vi "2.1 Interpret NMEA Sentence.vi"(11 "NMEA Sentence":string) -> ()   [LabVIEW 2011]
doc: "Interprets the NMEA 0813 sentences that we are using from our Airmar PB200 WeatherStation sensor.\nBy Jaime McCandless\nTODO: finish implementing NMEA sentences"
uses:
  2 Typedefs/Velocity.ctl
  2 Typedefs/apparent wind.ctl
  2 Typedefs/pitch and roll.ctl
  2 Globals/2 Global.vi
  <vilib>/regexp/Match Regular Expression.xnode
panel:
  out "Heading":dbl
  in  "UTC Time Zone":i32=-5
  out "Tab Control":T1(tab)
  out "GPS (GGA) Data":T2
  out "GPS (GLL) Data":T3
  out "UTC Time":timestamp
  out "Local Time":timestamp
  out "Lattitude (ddmm.mmmm)":dbl format="%_8g"
  out "Lattitude North/South":string
  out "Longitude (ddmm.mmmm)":dbl format="%_8g"
  out "Longitude East/West":string
  out "Speed over ground (knots)":dbl format="%_3g"
  out "Course over ground (degrees)":dbl format="%_4g"
  out "Magnetic Variation (degrees)":dbl format="%_4g"
  out "Variation East/West":string
  out "GPS (RMC) Data":T4 {"Course over ground (degrees)" format="%#.6g"; "Speed over ground (knots)" format="%#.6g"; "Magnetic Variation (degrees)" format="%#.6g"; "Longitude (ddmm.mmmm)" format="%#.6g"; "Lattitude (ddmm.mmmm)" format="%#.6g"}
  out "GPS Data Valid?":bool
  out "GPS (VTG) Data":T5
  out "Turn (ROT) Data":T6
  out "Wind (MWV) Data":T7
  out "Transducer (XDR) B Data":cluster{"Pitch (deg)":dbl, "Roll (deg)":dbl}
  out "Transducer (XDR) A Data":T8
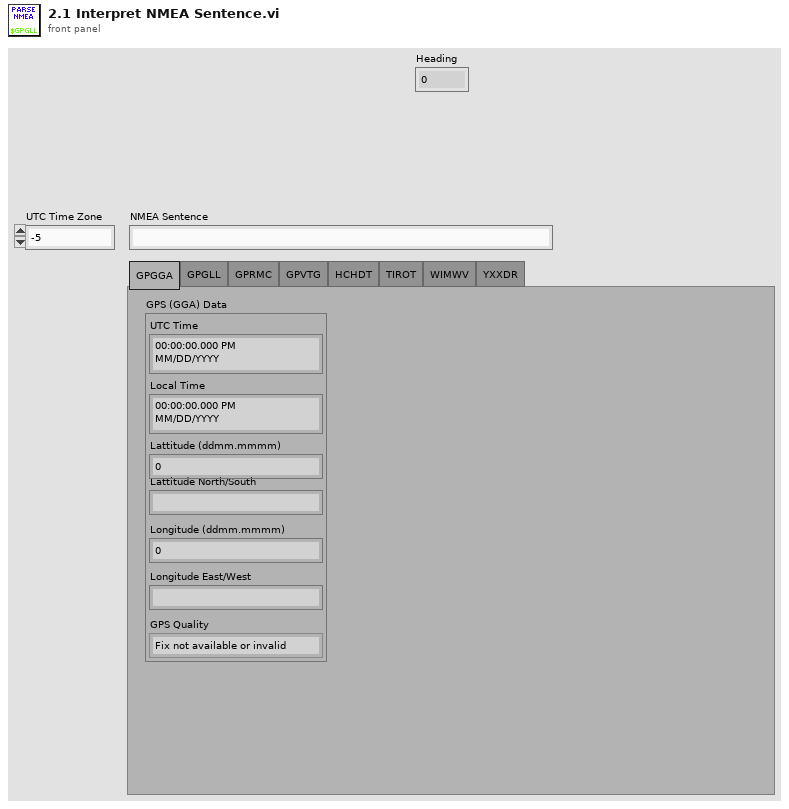
[diagram p1: front panel]
types:
  T1 = enum32{"GPGGA", "GPGLL", "GPRMC", "GPVTG", "HCHDT", "TIROT", "WIMWV", "YXXDR"}
  T2 = cluster{"UTC Time":timestamp, "Local Time":timestamp, "Lattitude (ddmm.mmmm)":dbl, "Lattitude North/South":string, "Longitude (ddmm.mmmm)":dbl, "Longitude East/West":string, "GPS Quality":enum16{"Fix not available or invalid", "GPS SPS Mode, fix valid", "Differential GPS, SPS Mode, fix valid", "GPS PPS Mode, fix valid", "Real Time Kinematic (RTK)", "Float RTK", "Estimated (dead reckoning) Mode", "Manual Input Mode", "Simulator Mode"}}
  T3 = cluster{"UTC Time":timestamp, "Local Time":timestamp, "Lattitude (ddmm.mmmm)":dbl, "Lattitude North/South":string, "Longitude (ddmm.mmmm)":dbl, "Longitude East/West":string, "GPS Mode":string, "GPS Data Valid?":bool}
  T4 = cluster{"UTC Time":timestamp, "Local Time":timestamp, "Lattitude (ddmm.mmmm)":dbl, "Lattitude North/South":string, "Longitude (ddmm.mmmm)":dbl, "Longitude East/West":string, "Magnetic Variation (degrees)":dbl, "Variation East/West":string, "Speed over ground (knots)":dbl, "Course over ground (degrees)":dbl}
  T5 = cluster{"Course Over Ground (True)":dbl, "Course Over Ground (Magnetic)":dbl, "Speed Over Ground (Knots)":dbl, "Speed Over Ground (km/hr)":dbl, "GPS Mode":string}
  T6 = cluster{"Rate of Turn (deg/min)":dbl, "Turn Rotation Data Valid?":bool}
  T7 = cluster{"Angle relative to boat (deg)":dbl, "Wind Data Valid?":bool, "Wind speed (knots)":dbl, "True (T) or Relative (R)":string}
  T8 = cluster{"Calc. Relative Wind Chill (degC)":dbl, "Calc. Theoretical Wind Chill (degC)":dbl, "Calc. Heat Index (degC)":dbl, "Meas. Barometric Pressure (bars)":dbl}
  T9 = cluster{"second":i32, "minute":i32, "hour":i32, "day of month":i32, "month":i32, "year":i32, "day of week":i32, "day of year":i32, "is DST":i32}
  T10 = typedef "Velocity.ctl" = cluster{"East":dbl, "North":dbl}
  T11 = typedef "apparent wind.ctl" = cluster{"Toward Fore":dbl, "Toward Starboard":dbl}
  T12 = typedef "pitch and roll.ctl" = cluster{"Pitch":dbl, "Roll":dbl}
  T13 = typedef "UTM Location.ctl" = cluster{"UTM Zone":dbl, "Hemisphere":enum16{"North", "South"}, "East":dbl, "North":dbl}
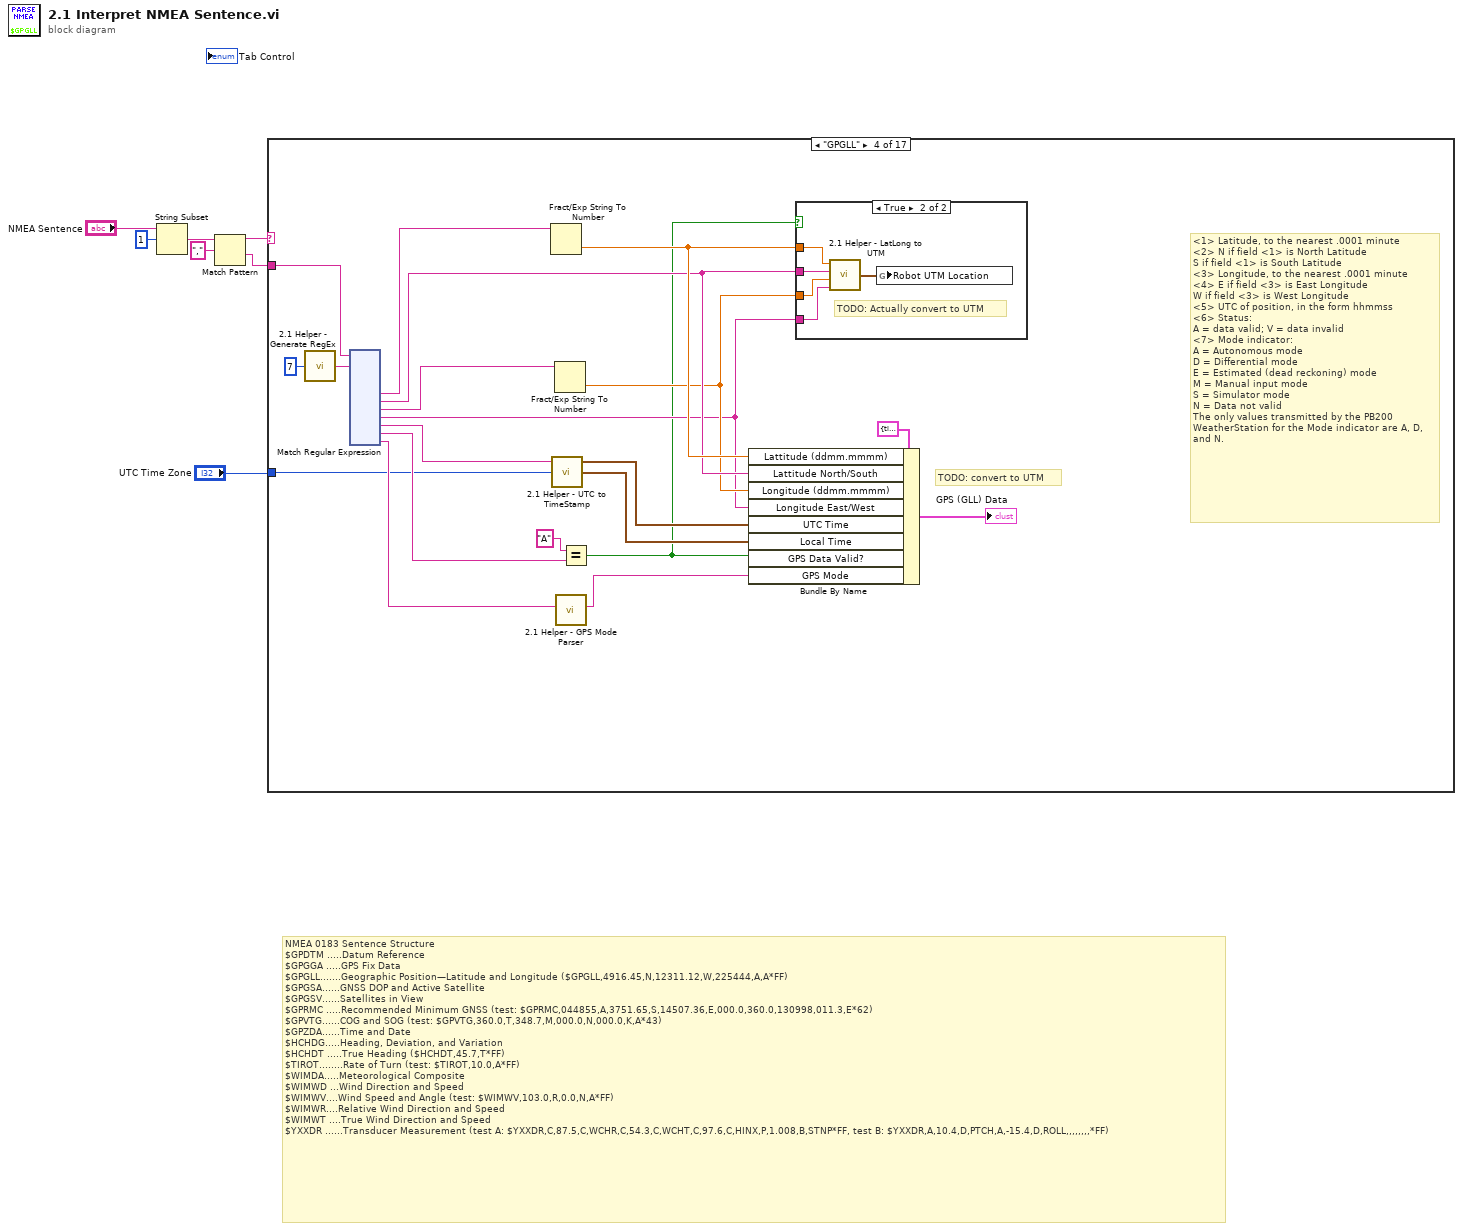
[diagram p0: block diagram]
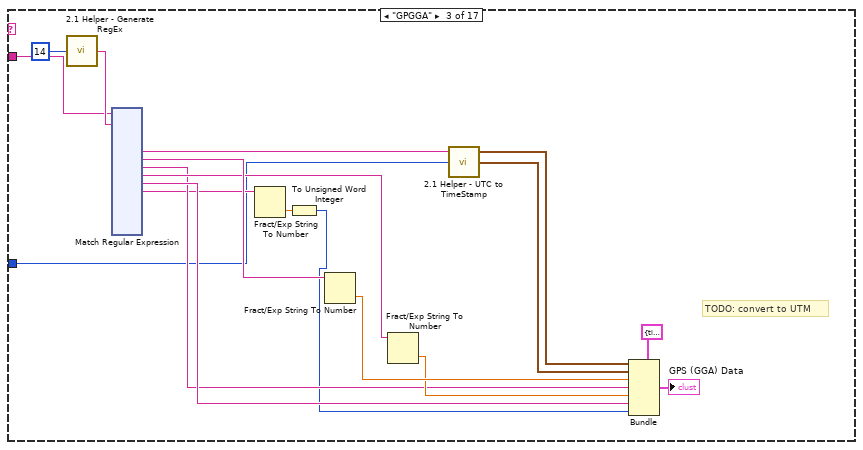
[diagram p4: hidden frame]
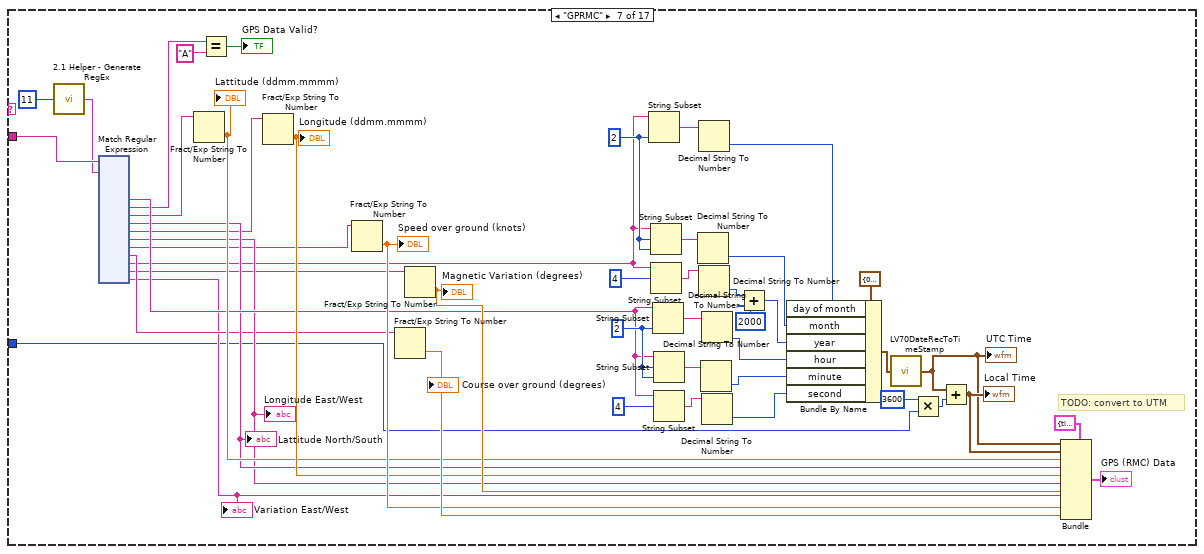
[diagram p8: hidden frame]
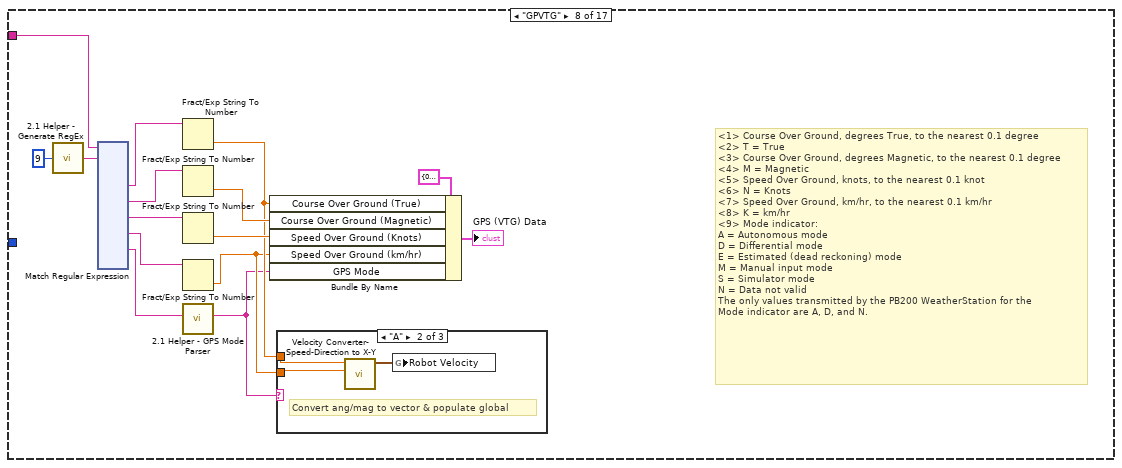
[diagram p9: hidden frame]
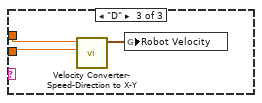
[diagram p11: hidden frame]
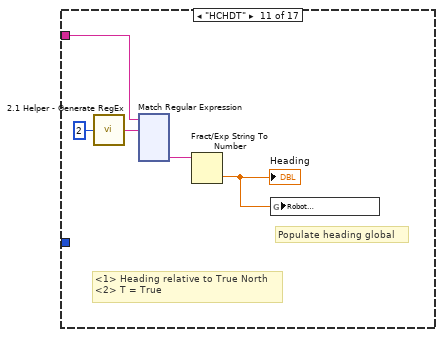
[diagram p14: hidden frame]
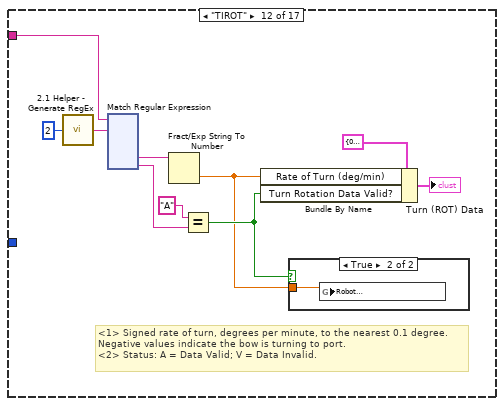
[diagram p15: hidden frame]
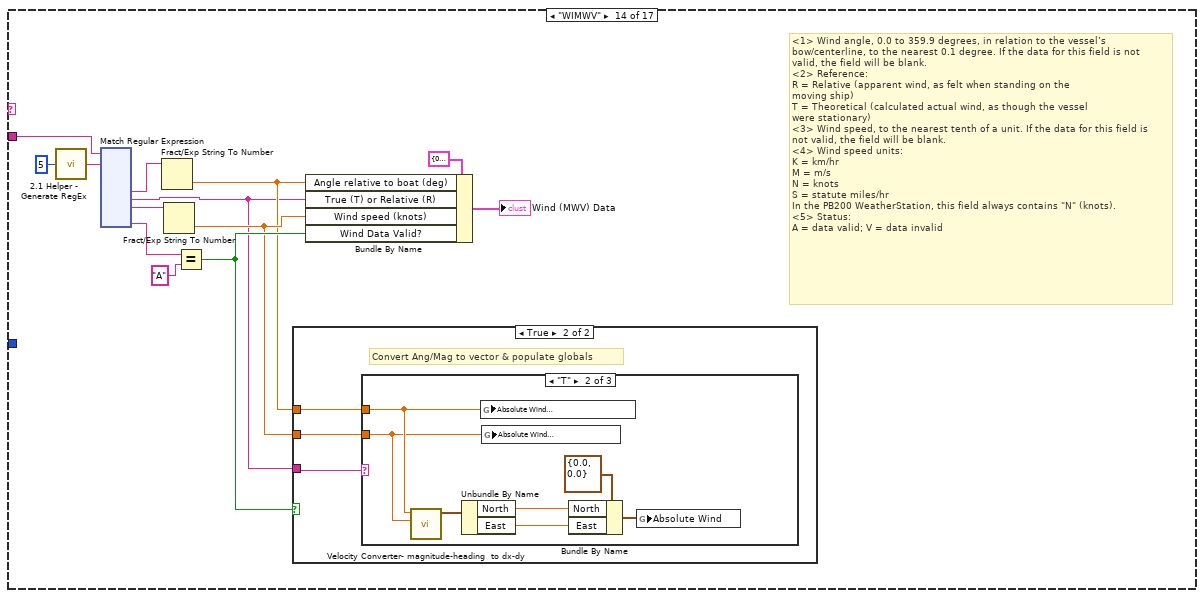
[diagram p18: hidden frame]
diagram:
  # "NMEA 0183 Sentence Structure\n$GPDTM .....Datum Reference\n$GPGGA .....GPS Fix Data\n$GPGLL.......Geographic Position—Latitude and Longitude ($GPGLL,4916.45,N,12311.12,W,225444,A,A*FF)\n$GPGSA......GNSS DOP and Active Satellite\n$GPGSV......Satellites in View\n$GPRMC .....Recommended Minimum GNSS (test: $GPRMC,044855,A,3751.65,S,14507.36,E,000.0,360.0,130998,011.3,E*62)\n$GPVTG......COG and SOG (test: $GPVTG,360.0,T,348.7,M,000.0,N,000.0,K,A*43)\n$GPZDA......Time and Date\n$HCHDG.....Heading, Deviation, and Variation\n$HCHDT .....True Heading ($HCHDT,45.7,T*FF)\n$TIROT........Rate of Turn (test: $TIROT,10.0,A*FF)\n$WIMDA.....Meteorological Composite\n$WIMWD ...Wind Direction and Speed\n$WIMWV....Wind Speed and Angle (test: $WIMWV,103.0,R,0.0,N,A*FF)\n$WIMWR....Relative Wind Direction and Speed\n$WIMWT ....True Wind Direction and Speed\n$YXXDR ......Transducer Measurement (test A: $YXXDR,C,87.5,C,WCHR,C,54.3,C,WCHT,C,97.6,C,HINX,P,1.008,B,STNP*FF, test B: $YXXDR,A,10.4,D,PTCH,A,-15.4,D,ROLL,,,,,,,,*FF)"
  n1 = String Subset(string="NMEA Sentence", offset (0)=1) -> (substring=w4:string)  [unwired: 1 in]
  n2 = Match Pattern(string=w4, regular expression=",") -> (before substring=w5:string, after substring=w6:string)  [unwired: 1 in, 2 out]
  n3 = case shown="\"GPGLL\"" w5 {
    tunnel: w6 -> [_ _ w23 w163 _ _ w307 w476 _ _ w610 w732 _ w859 _ _ w1003]
    tunnel: "UTC Time Zone" -> [_ _ w8 w155 _ _ w293 _ _ _ _ _ _ _ _ _ _]
    frame "", Default {
    }
    frame "GPDTM" {
    }
    frame "GPGGA" {
      # "TODO: convert to UTM"
      n4 = call "2.1 Helper - Generate RegEx.vi"("# Datums"=14) -> ("RegEx"=w24:string)
      n5 = xnode "Match Regular Expression"("input string"=w23, "regular expression"=w24) -> ("submatch 1"=w11:string, "submatch 2"=w19:string, "submatch 3"=w16:string, "submatch 4"=w18:string, "submatch 5"=w17:string, "submatch 6"=w15:string)  [unwired: 4 in, 10 out]
      n6 = Fract/Exp String To Number(string=w15) -> (number=w14:dbl)  [unwired: 3 in, 1 out]
      n7 = To Unsigned Word Integer(number=w14) -> (unsigned 16bit integer=w13:u16)
      n8 = Fract/Exp String To Number(string=w19) -> (number=w22:dbl)  [unwired: 3 in, 1 out]
      n9 = Fract/Exp String To Number(string=w18) -> (number=w21:dbl)  [unwired: 3 in, 1 out]
      n10 = call "2.1 Helper - UTC to TimeStamp.vi"("UTC Time Zone in"=w8, "UTC (hhmmss)"=w11) -> ("Local Time"=w9:timestamp, "UTC Time"=w10:timestamp)  [unwired: 2 in]
      n11 = Bundle(cluster=T2 {"UTC Time"=timestamp(0 s since 1904-01-01), "Local Time"=timestamp(0 s since 1904-01-01), "Lattitude (ddmm.mmmm)"=0.0, "Lattitude North/South"="", "Longitude (ddmm.mmmm)"=0.0, "Longitude East/West"="", "GPS Quality"=enum."GPS SPS Mode, fix valid"} ("Cluster"), "UTC Time"=w10, "Local Time"=w9, "Lattitude (ddmm.mmmm)"=w22, "Lattitude North/South"=w16, "Longitude (ddmm.mmmm)"=w21, "Longitude East/West"=w17, "GPS Quality"=w13) -> (→"GPS (GGA) Data":T2)
    }
    frame "GPGLL" {
      # "<1> Latitude, to the nearest .0001 minute\n<2> N if field <1> is North Latitude\nS if field <1> is South Latitude\n<3> Longitude, to the nearest .0001 minute\n<4> E if field <3> is East Longitude\nW if field <3> is West Longitude\n<5> UTC of position, in the form hhmmss\n<6> Status:\nA = data valid; V = data invalid\n<7> Mode indicator:\nA = Autonomous mode\nD = Differential mode\nE = Estimated (dead reckoning) mode\nM = Manual input mode\nS = Simulator mode\nN = Data not valid\nThe only values transmitted by the PB200 WeatherStation for the Mode indicator are A, D, and N."
      # "TODO: convert to UTM"
      n12 = call "2.1 Helper - Generate RegEx.vi"("# Datums"=7) -> ("RegEx"=w167:string)
      n13 = xnode "Match Regular Expression"("input string"=w163, "regular expression"=w167) -> ("submatch 1"=w166:string, "submatch 2"=w152:string, "submatch 3"=w165:string, "submatch 4"=w150:string, "submatch 5"=w162:string, "submatch 6"=w158:string, "submatch 7"=w164:string)  [unwired: 4 in, 5 out]
      n14 = Fract/Exp String To Number(string=w166) -> (number=w153:dbl)  [unwired: 3 in, 1 out]
      n15 = call "2.1 Helper - UTC to TimeStamp.vi"("UTC Time Zone in"=w155, "UTC (hhmmss)"=w162) -> ("Local Time"=w157:timestamp, "UTC Time"=w156:timestamp)  [unwired: 2 in]
      n16 = Fract/Exp String To Number(string=w165) -> (number=w151:dbl)  [unwired: 3 in, 1 out]
      n17 = call "2.1 Helper - GPS Mode Parser.vi"("GPS Mode (Char)"=w164) -> ("GPS Mode (Description)"=w160:string)  [unwired: 6 in]
      n18 = Equal?(x="A" ("y"), y=w158) -> (x = y?=w149:bool)
      n19 = Bundle By Name(cluster=T3 {"UTC Time"=timestamp(0 s since 1904-01-01), "Local Time"=timestamp(0 s since 1904-01-01), "Lattitude (ddmm.mmmm)"=0.0, "Lattitude North/South"="", "Longitude (ddmm.mmmm)"=0.0, "Longitude East/West"="", "GPS Mode"="", "GPS Data Valid?"=FALSE} ("Cluster"), "Lattitude (ddmm.mmmm)"=w153, "Lattitude North/South"=w152, "Longitude (ddmm.mmmm)"=w151, "Longitude East/West"=w150, "UTC Time"=w156, "Local Time"=w157, "GPS Data Valid?"=w149, "GPS Mode"=w160) -> (→"GPS (GLL) Data":T3)
      n20 = case shown="True" w149 {
        tunnel: w153 -> [_ w172]
        tunnel: w152 -> [_ w171]
        tunnel: w151 -> [_ w170]
        tunnel: w150 -> [_ w169]
        frame False {
        }
        frame True {
          # "TODO: Actually convert to UTM"
          n21 = call "2.1 Helper - LatLong to UTM.vi"("East/West"=w169, "Longitude"=w170, "North/South"=w171, "Latitude"=w172) -> ("Robot UTM Location"=w173:T13)
          n22 = global write "2 Global.vi" "Robot UTM Location"(w173) -> ()
        }
      }
    }
    frame "GPGSA" {
    }
    frame "GPGSV" {
    }
    frame "GPRMC" {
      w325 = 2 ("length (rest)")
      w315 = 2 ("length (rest)")
      # "TODO: convert to UTM"
      n23 = call "2.1 Helper - Generate RegEx.vi"("# Datums"=11) -> ("RegEx"=w295:string)
      n24 = xnode "Match Regular Expression"("input string"=w307, "regular expression"=w295) -> ("submatch 1"=w306:string, "submatch 2"=w305:string, "submatch 3"=w304:string, "submatch 4"=w303:string, "submatch 5"=w302:string, "submatch 6"=w301:string, "submatch 7"=w300:string, "submatch 8"=w299:string, "submatch 9"=w298:string, "submatch 10"=w297:string, "submatch 11"=w296:string)  [unwired: 4 in, 5 out]
      "Lattitude North/South" <- w303
      "Longitude East/West" <- w301
      "Variation East/West" <- w296
      n25 = Fract/Exp String To Number(string=w304) -> (number=w334:dbl)  [unwired: 3 in, 1 out]
      "Lattitude (ddmm.mmmm)" <- w334
      n26 = Equal?(x=w305, y="A") -> (x = y?=→"GPS Data Valid?":bool)
      n27 = Fract/Exp String To Number(string=w302) -> (number=w335:dbl)  [unwired: 3 in, 1 out]
      "Longitude (ddmm.mmmm)" <- w335
      n28 = Fract/Exp String To Number(string=w300) -> (number=w337:dbl)  [unwired: 3 in, 1 out]
      "Speed over ground (knots)" <- w337
      n29 = Fract/Exp String To Number(string=w299) -> (number=w338:dbl)  [unwired: 3 in, 1 out]
      "Course over ground (degrees)" <- w338
      n30 = Fract/Exp String To Number(string=w297) -> (number=w336:dbl)  [unwired: 3 in, 1 out]
      "Magnetic Variation (degrees)" <- w336
      n31 = String Subset(string=w298, length (rest)=w325) -> (substring=w326:string)  [unwired: 1 in]
      n32 = String Subset(string=w298, offset (0)=w325, length (rest)=w325) -> (substring=w324:string)
      n33 = String Subset(string=w298, offset (0)=4) -> (substring=w322:string)  [unwired: 1 in]
      n34 = String Subset(string=w306, length (rest)=w315) -> (substring=w311:string)  [unwired: 1 in]
      n35 = String Subset(string=w306, offset (0)=w315, length (rest)=w315) -> (substring=w317:string)
      n36 = String Subset(string=w306, offset (0)=4) -> (substring=w319:string)  [unwired: 1 in]
      n37 = Decimal String To Number(string=w324) -> (number=w328:i32)  [unwired: 2 in, 1 out]
      n38 = Decimal String To Number(string=w326) -> (number=w327:i32)  [unwired: 2 in, 1 out]
      n39 = Decimal String To Number(string=w322) -> (number=w329:i32)  [unwired: 2 in, 1 out]
      n40 = Decimal String To Number(string=w317) -> (number=w316:i32)  [unwired: 2 in, 1 out]
      n41 = Decimal String To Number(string=w311) -> (number=w314:i32)  [unwired: 2 in, 1 out]
      n42 = Decimal String To Number(string=w319) -> (number=w320:i32)  [unwired: 2 in, 1 out]
      n43 = Add(x=w329, y=2000) -> (x+y=w331:i32)
      n44 = Bundle By Name(cluster=T9 {"second"=0, "minute"=0, "hour"=0, "day of month"=0, "month"=0, "year"=0, "day of week"=0, "day of year"=0, "is DST"=0} ("date time rec"), "day of month"=w327, "month"=w328, "year"=w331, "hour"=w314, "minute"=w316, "second"=w320) -> (w312:T9)
      n45 = call <vilib>:"LV70DateRecToTimeStamp.vi"("date time rec"=w312) -> ("Time Stamp"=w332:timestamp)
      "UTC Time" <- w332
      n46 = Multiply(x=3600 ("number"), y=w293) -> (x*y=w294:i32)
      n47 = Add(x=w332, y=w294) -> (x+y=w333:timestamp)
      "Local Time" <- w333
      n48 = Bundle(cluster=T4 {"UTC Time"=timestamp(0 s since 1904-01-01), "Local Time"=timestamp(0 s since 1904-01-01), "Lattitude (ddmm.mmmm)"=0.0, "Lattitude North/South"="", "Longitude (ddmm.mmmm)"=0.0, "Longitude East/West"="", "Magnetic Variation (degrees)"=0.0, "Variation East/West"="", "Speed over ground (knots)"=0.0, "Course over ground (degrees)"=0.0} ("Cluster"), "UTC Time"=w332, "Local Time"=w333, "Lattitude (ddmm.mmmm)"=w334, "Lattitude North/South"=w303, "Longitude (ddmm.mmmm)"=w335, "Longitude East/West"=w301, "Magnetic Variation (degrees)"=w336, "Variation East/West"=w296, "Speed over ground (knots)"=w337, "Course over ground (degrees)"=w338) -> (→"GPS (RMC) Data":T4)
    }
    frame "GPVTG" {
      # "<1> Course Over Ground, degrees True, to the nearest 0.1 degree\n<2> T = True\n<3> Course Over Ground, degrees Magnetic, to the nearest 0.1 degree\n<4> M = Magnetic\n<5> Speed Over Ground, knots, to the nearest 0.1 knot\n<6> N = Knots\n<7> Speed Over Ground, km/hr, to the nearest 0.1 km/hr\n<8> K = km/hr\n<9> Mode indicator:\nA = Autonomous mode\nD = Differential mode\nE = Estimated (dead reckoning) mode\nM = Manual input mode\nS = Simulator mode\nN = Data not valid\nThe only values transmitted by the PB200 WeatherStation for the\nMode indicator are A, D, and N."
      n49 = call "2.1 Helper - Generate RegEx.vi"("# Datums"=9) -> ("RegEx"=w477:string)
      n50 = xnode "Match Regular Expression"("input string"=w476, "regular expression"=w477) -> ("submatch 1"=w473:string, "submatch 3"=w472:string, "submatch 5"=w470:string, "submatch 7"=w468:string, "submatch 9"=w467:string)  [unwired: 4 in, 11 out]
      n51 = Fract/Exp String To Number(string=w473) -> (number=w466:dbl)  [unwired: 3 in, 1 out]
      n52 = Fract/Exp String To Number(string=w472) -> (number=w471:dbl)  [unwired: 3 in, 1 out]
      n53 = Fract/Exp String To Number(string=w470) -> (number=w469:dbl)  [unwired: 3 in, 1 out]
      n54 = Fract/Exp String To Number(string=w468) -> (number=w465:dbl)  [unwired: 3 in, 1 out]
      n55 = call "2.1 Helper - GPS Mode Parser.vi"("GPS Mode (Char)"=w467) -> ("GPS Mode (Description)"=w464:string)  [unwired: 6 in]
      n56 = Bundle By Name(cluster=T5 {"Course Over Ground (True)"=0.0, "Course Over Ground (Magnetic)"=0.0, "Speed Over Ground (Knots)"=0.0, "Speed Over Ground (km/hr)"=0.0, "GPS Mode"=""} ("GPS (VTG) Data 2"), "Course Over Ground (True)"=w466, "Course Over Ground (Magnetic)"=w471, "Speed Over Ground (Knots)"=w469, "Speed Over Ground (km/hr)"=w465, "GPS Mode"=w464) -> (→"GPS (VTG) Data":T5)
      n57 = case shown="\"A\"" w464 {
        tunnel: w466 -> [_ w481 w484]
        tunnel: w465 -> [_ w480 w483]
        frame "N", Default {
          # "Data not valid"
        }
        frame "A" {
          # "Convert ang/mag to vector & populate global"
          n58 = call "Velocity Converter- Speed-Direction to X-Y.vi"("Speed"=w480, "Heading"=w481) -> ("Velocity Out"=w479:T10)  [unwired: 9 in]
          n59 = global write "2 Global.vi" "Robot Velocity"(w479) -> ()
        }
        frame "D" {
          n60 = call "Velocity Converter- Speed-Direction to X-Y.vi"("Speed"=w483, "Heading"=w484) -> ("Velocity Out"=w482:T10)  [unwired: 9 in]
          n61 = global write "2 Global.vi" "Robot Velocity"(w482) -> ()
        }
      }
    }
    frame "GPZDA" {
    }
    frame "HCHDG " {
    }
    frame "HCHDT" {
      # "Populate heading global"
      # "<1> Heading relative to True North\n<2> T = True"
      n62 = call "2.1 Helper - Generate RegEx.vi"("# Datums"=2) -> ("RegEx"=w611:string)
      n63 = xnode "Match Regular Expression"("input string"=w610, "regular expression"=w611) -> ("submatch 1"=w609:string)  [unwired: 4 in, 5 out]
      n64 = Fract/Exp String To Number(string=w609) -> (number=w608:dbl)  [unwired: 3 in, 1 out]
      "Heading" <- w608
      n65 = global write "2 Global.vi" "Robot\nHeading"(w608) -> ()
    }
    frame "TIROT" {
      # "<1> Signed rate of turn, degrees per minute, to the nearest 0.1 degree.\nNegative values indicate the bow is turning to port.\n<2> Status: A = Data Valid; V = Data Invalid."
      n66 = call "2.1 Helper - Generate RegEx.vi"("# Datums"=2) -> ("RegEx"=w734:string)
      n67 = xnode "Match Regular Expression"("input string"=w732, "regular expression"=w734) -> ("submatch 1"=w733:string, "submatch 2"=w728:string)  [unwired: 4 in, 5 out]
      n68 = Fract/Exp String To Number(string=w733) -> (number=w726:dbl)  [unwired: 3 in, 1 out]
      n69 = Equal?(x="A" ("y"), y=w728) -> (x = y?=w727:bool)
      n70 = Bundle By Name(cluster=T6 {"Rate of Turn (deg/min)"=0.0, "Turn Rotation Data Valid?"=TRUE} ("Turn (ROT) Data 2"), "Rate of Turn (deg/min)"=w726, "Turn Rotation Data Valid?"=w727) -> (→"Turn (ROT) Data":T6)
      n71 = case shown="True" w727 {
        tunnel: w726 -> [_ w736]
        frame False {
        }
        frame True {
          n72 = global write "2 Global.vi" "Robot\nRate of Turn"(w736) -> ()
        }
      }
    }
    frame "WIMDA" {
    }
    frame "WIMWV" {
      # "<1> Wind angle, 0.0 to 359.9 degrees, in relation to the vessel’s\nbow/centerline, to the nearest 0.1 degree. If the data for this field is not\nvalid, the field will be blank.\n<2> Reference:\nR = Relative (apparent wind, as felt when standing on the\nmoving ship)\nT = Theoretical (calculated actual wind, as though the vessel\nwere stationary)\n<3> Wind speed, to the nearest tenth of a unit. If the data for this field is\nnot valid, the field will be blank.\n<4> Wind speed units:\nK = km/hr\nM = m/s\nN = knots\nS = statute miles/hr\nIn the PB200 WeatherStation, this field always contains \"N\" (knots).\n<5> Status:\nA = data valid; V = data invalid"
      n73 = call "2.1 Helper - Generate RegEx.vi"("# Datums"=5) -> ("RegEx"=w862:string)
      n74 = xnode "Match Regular Expression"("input string"=w859, "regular expression"=w862) -> ("submatch 1"=w861:string, "submatch 2"=w851:string, "submatch 3"=w856:string, "submatch 5"=w855:string)  [unwired: 4 in, 6 out]
      n75 = Fract/Exp String To Number(string=w861) -> (number=w852:dbl)  [unwired: 3 in, 1 out]
      n76 = Fract/Exp String To Number(string=w856) -> (number=w853:dbl)  [unwired: 3 in, 1 out]
      n77 = Equal?(x=w855, y="A") -> (x = y?=w854:bool)
      n78 = case shown="True" w854 {
        tunnel: w853 -> [_ w866]
        tunnel: w852 -> [_ w865]
        tunnel: w851 -> [_ w864]
        frame False {
        }
        frame True {
          # "Convert Ang/Mag to vector & populate globals"
          n79 = case shown="\"T\"" w864 {
            tunnel: w866 -> [_ w868 w874]
            tunnel: w865 -> [_ w869 w875]
            frame "\u0000", Default {
            }
            frame "T" {
              n80 = call "Velocity Converter- magnitude-heading  to dx-dy.vi"("Magnitude"=w868, "Heading"=w869) -> ("Vector Out"=w873:T10)  [unwired: 9 in]
              n81 = Unbundle By Name(w873) -> ("North"=w871:dbl, "East"=w870:dbl)
              n82 = global write "2 Global.vi" "Absolute Wind\nDirection"(w869) -> ()
              n83 = global write "2 Global.vi" "Absolute Wind\nSpeed"(w868) -> ()
              n84 = Bundle By Name(cluster=T10 {"East"=0.0, "North"=0.0} ("Absolute Wind"), "North"=w871, "East"=w870) -> (w872:T10)
              n85 = global write "2 Global.vi" "Absolute Wind"(w872) -> ()
            }
            frame "R" {
              n86 = call "Velocity Converter- magnitude-heading  to dx-dy.vi"("Magnitude"=w874, "Heading"=w875) -> ("Vector Out"=w876:T10)  [unwired: 9 in]
              n87 = Unbundle By Name(w876) -> ("North"=w879:dbl, "East"=w880:dbl)
              n88 = global write "2 Global.vi" "Apparent Wind\nDirection"(w875) -> ()
              n89 = global write "2 Global.vi" "Apparent Wind\nSpeed"(w874) -> ()
              n90 = Bundle By Name(cluster=T11 {"Toward Fore"=0.0, "Toward Starboard"=0.0} ("Apparent Wind"), "Toward Fore"=w879, "Toward Starboard"=w880) -> (w878:T11)
              n91 = global write "2 Global.vi" "Apparent Wind"(w878) -> ()
            }
          }
        }
      }
      n92 = Bundle By Name(cluster=T7 {"Angle relative to boat (deg)"=0.0, "Wind Data Valid?"=TRUE, "Wind speed (knots)"=0.0, "True (T) or Relative (R)"=""} ("Wind (MWV) Data 2"), "Angle relative to boat (deg)"=w852, "True (T) or Relative (R)"=w851, "Wind speed (knots)"=w853, "Wind Data Valid?"=w854) -> (→"Wind (MWV) Data":T7)
    }
    frame "WIMWR" {
    }
    frame "WIMWT" {
    }
    frame "YXXDR" {
      n93 = call "2.1 Helper - Generate RegEx.vi"("# Datums"=16) -> ("RegEx"=w1005:string)
      n94 = xnode "Match Regular Expression"("input string"=w1003, "regular expression"=w1005) -> ("submatch 1"=w1002:string, "submatch 2"=w1001:string, "submatch 6"=w1000:string, "submatch 10"=w999:string, "submatch 14"=w998:string)  [unwired: 4 in, 16 out]
      n95 = case shown="\"C\"" w1002 {
        tunnel: w1001 -> [_ w1011 w1021]
        tunnel: w1000 -> [_ w1010 w1020]
        tunnel: w999 -> [_ _ w1018]
        tunnel: w998 -> [_ _ w1019]
        frame "", Default {
        }
        frame "A" {
          # "TYPE B:\n<1> A = angular displacement\n<2> Pitch: oscillation of vessel about its latitudinal axis. Bow moving up is positive. Value reported to the nearest 0.1 degree.\n<3> D = degrees\n<4> PTCH (ID indicating pitch of vessel)\n<5> A = angular displacement\n<6> Roll: oscillation of vessel about its longitudinal axis. Roll to the starboard is positive. Value reported to the nearest 0.1 degree.\n<7> D = degrees\n<8> ROLL (ID indicating roll of vessel)\n<9> Not used\n<10> Not used\n<11> Not used\n<12> Not used\n<13> Not used\n<14> Not used\n<15> Not used\n<16> Not used"
          n96 = Fract/Exp String To Number(string=w1011) -> (number=w1007:dbl)  [unwired: 3 in, 1 out]
          n97 = Fract/Exp String To Number(string=w1010) -> (number=w1006:dbl)  [unwired: 3 in, 1 out]
          n98 = Bundle By Name(cluster=cluster{"Pitch (deg)":dbl, "Roll (deg)":dbl} {"Pitch (deg)"=103.0, "Roll (deg)"=103.0} ("Transducer (XDR) B Data 2"), "Pitch (deg)"=w1007, "Roll (deg)"=w1006) -> (→"Transducer (XDR) B Data":cluster{"Pitch (deg)":dbl, "Roll (deg)":dbl})
          n99 = Bundle By Name(cluster=T12 {"Pitch"=0.0, "Roll"=0.0} ("Robot Pitch/Roll"), "Pitch"=w1007, "Roll"=w1006) -> (w1008:T12)
          n100 = global write "2 Global.vi" "Robot Pitch/Roll"(w1008) -> ()
        }
        frame "C" {
          # "TYPE A:\n<1> C = temperature\n<2> Calculated “relative” wind chill temperature, degrees Celsius, to the nearest 0.1 degree\n<3> C = degrees C\n<4> WCHR (ID indicating relative wind chill)\n<5> C = temperature\n<6> Calculated “theoretical” wind chill temperature, degrees Celsius, to the nearest 0.1 degree\n<7> C = degrees C\n<8> WCHT (ID indicating theoretical wind chill)\n<9> C = temperature\n<10> Calculated heat index, degrees Celsius, to the nearest 0.1 degree (this field left blank by WeatherStation)\n<11> C = degrees C\n<12> HINX (ID indicating heat index)\n<13> P = pressure\n<14> Actual measured barometric pressure, or \"station pressure\", bars, to the nearest 0.001 bar\n<15> B = bars\n<16> STNP (ID indicating station pressure)"
          n101 = Fract/Exp String To Number(string=w1021) -> (number=w1017:dbl)  [unwired: 3 in, 1 out]
          n102 = Fract/Exp String To Number(string=w1020) -> (number=w1016:dbl)  [unwired: 3 in, 1 out]
          n103 = Fract/Exp String To Number(string=w1018) -> (number=w1015:dbl)  [unwired: 3 in, 1 out]
          n104 = Fract/Exp String To Number(string=w1019) -> (number=w1014:dbl)  [unwired: 3 in, 1 out]
          n105 = Bundle By Name(cluster=T8 {"Calc. Relative Wind Chill (degC)"=0.0, "Calc. Theoretical Wind Chill (degC)"=0.0, "Calc. Heat Index (degC)"=0.0, "Meas. Barometric Pressure (bars)"=0.0} ("Transducer (XDR) A Data 2"), "Calc. Relative Wind Chill (degC)"=w1017, "Calc. Theoretical Wind Chill (degC)"=w1016, "Calc. Heat Index (degC)"=w1015, "Meas. Barometric Pressure (bars)"=w1014) -> (→"Transducer (XDR) A Data":T8)
        }
      }
    }
  }
